vi "Read Data.vi"(8 "error in (no error)":errorcluster, 11 "Terminal in":refnum<class "Terminal.lvclass">) -> (0 "error out":errorcluster, 3 "Terminal out":refnum<class "Terminal.lvclass">)   [LabVIEW 2020, in "Terminal.lvlib" / "Terminal.lvclass"]
uses:
  Terminal.lvclass
  Terminal.lvclass/Terminal.ctl
  <vilib>/IlluminatedG/lv-stream/Connection/Connection.lvclass
  <vilib>/IlluminatedG/lv-stream/stream/Stream.lvclass
panel:
  out "Data":string
  in  "Count":i32
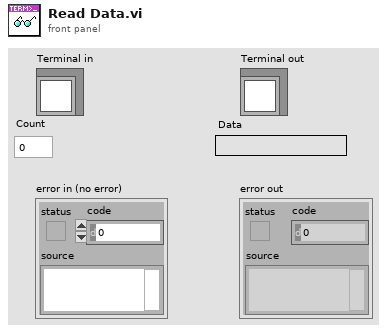
[diagram p1: front panel]
types:
  T1 = typedef "Terminal.lvlib/Terminal.lvclass/Ref Data.ctl" = cluster{"Connection":refnum<class "Connection.lvclass">, "Font":cluster{"Font Name:":string, "Size":i16, "Strikeout?":bool, "Italic?":bool, "Underline?":bool, "Outline?":bool, "Shadow?":bool, "Bold?":bool}, "Color Scheme":T2, "Default FG":T3, "Default BG":T3, "History Length":i32, "History Queue":refnum<queue>, "Read Loop Running":bool}
  T2 = typedef "Terminal.lvlib/Terminal.lvclass/Color Scheme.ctl" = cluster{"Black":u32, "Red":u32, "Green":u32, "Yellow":u32, "Blue":u32, "Magenta":u32, "Cyan":u32, "White":u32, "Bright Black":u32, "Bright Red":u32, "Bright Green":u32, "Bright Yellow":u32, "Bright Blue":u32, "Bright Magenta":u32, "Bright Cyan":u32, "Bright White":u32}
  T3 = typedef "Terminal.lvlib/Terminal.lvclass/Color.ctl" = i8
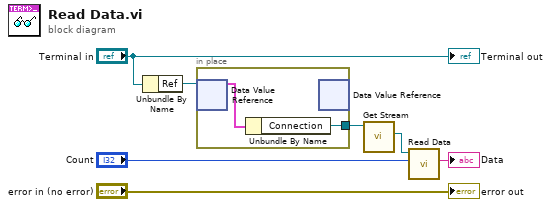
[diagram p0: block diagram]
diagram:
  n1 = Unbundle By Name("Terminal in") -> ("Ref"=w6:refnum<data-value>)
  n2 = in-place {
    in-place-border: [w8] -> w5
    n3 = in-place-dvr #1(w6) -> (w9:T1)  [unwired: 1 out]
    n4 = Unbundle By Name(w9) -> ("Connection"=w8:refnum<class "Connection.lvclass">)
    n5 = in-place-dvr #1() -> ()  [unwired: 1 in, 2 out]
  }
  n6 = call-dynamic "Get Stream.vi"("Connection in"=w5) -> ("Stream"=w3:refnum<class "Stream.lvclass">)  [unwired: 8 in, 2 out]
  n7 = call-dynamic "Read Data.vi"("Count"="Count", "Stream in"=w3) -> ("Data"=→"Data":string)  [unwired: 7 in, 2 out]
  "error out" <- "error in (no error)"
  "Terminal out" <- "Terminal in"
